vi "Trav_move_above_height.vi"(0 "Mode":T3, 1 "Extra Command String":string, 3 "Home Z":T1, 5 "New Position":sgl[](array[numeric])=[0.0, 0.0, 0.0] format="%.2f", 9 "Backlash Compensation?":bool=TRUE, 11 "Simulate/Run":T2, 12 "Row Number":i32=11, 13 "Currently on Point":i32=11, 14 "Last Part of Move?":bool=TRUE) -> (4 "Trav Position achieved":sgl[](array[numeric]) format="%.2f", 6 "Error from Traverse named":string, 15 "Error String":string)   [LabVIEW 2015]
uses:
  Trav_mode.ctl
  Controls/User_Specific_mode.ctl
  Controls/Home.ctl
  Controls/Tunnel_Coordinates.ctl
  Globals/Trav_pos_global.vi
  Globals/Extra_Commands_Global.vi
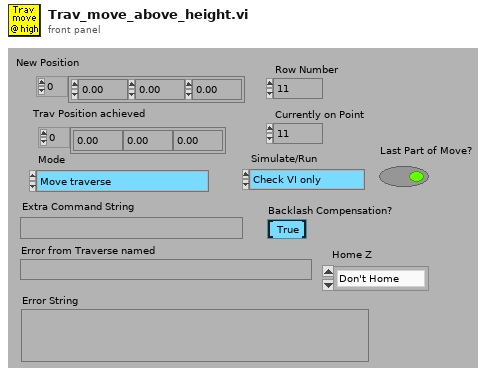
[diagram p1: front panel]
types:
  T1 = typedef "Home.ctl" = enum16{"Don't Home", "Home  +X", "Home  -X", "Home  +Y", "Home  -Y", "Home  +Z", "Home  -Z"}
  T2 = typedef "User_Specific_mode.ctl" = enum16{"Check VI only", "Run VI"}
  T3 = typedef "Trav_mode.ctl" = enum16{"Move traverse", "Read traverse position", "Teach Position"}
  T4 = typedef "Tunnel_Coordinates.ctl" = enum16{"Work in Tunnel Coordinates", "Work in Model Coordinates"}
  T5 = enum16{"To Traverse Coordinates", "To User Coordinates"}
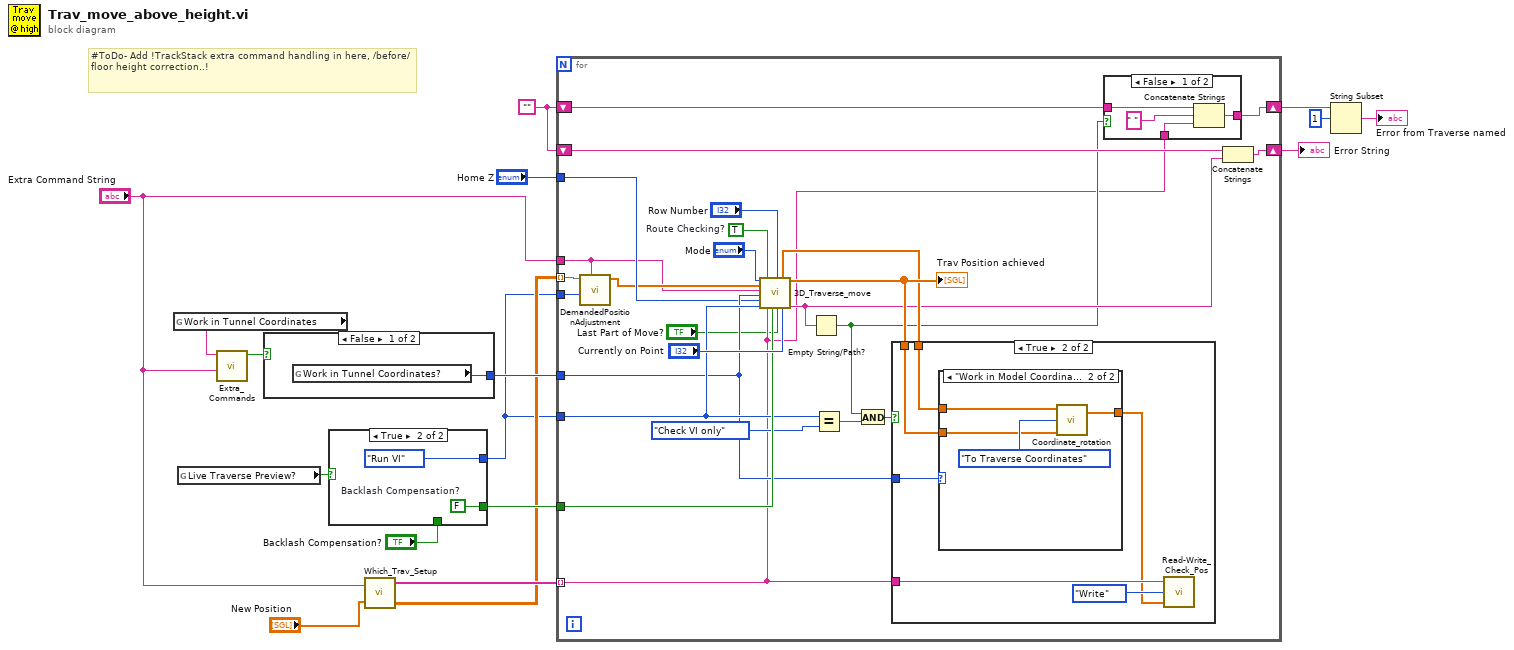
[diagram p0: block diagram]
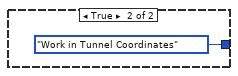
[diagram p5: hidden frame]
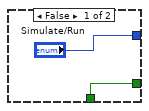
[diagram p6: hidden frame]
diagram:
  w10 = ""
  # "#ToDo- Add !TrackStack extra command handling in here, /before/ floor height correction..!"
  n1 = global read "Extra_Commands_Global.vi" "Work in Tunnel Coordinates"() -> (w14:string)
  n2 = global read "Trav_pos_global.vi" "Live Traverse Preview?"() -> (w17:bool)
  n3 = call "Extra_Commands.vi"("String to Search"="Extra Command String", "Command"=w14) -> ("Command Found"=w13:bool)  [unwired: 1 in, 4 out]
  n4 = case shown="False" w13 {
    tunnel: [w18 Tunnel_Coordinates."Work in Tunnel Coordinates" ("Work in Tunnel Coordinates?")] -> w12
    frame False {
      n5 = global read "Trav_pos_global.vi" "Work in Tunnel Coordinates?"() -> (w18:T4)
    }
    frame True {
    }
  }
  n6 = case shown="True" w17 {
    tunnel: ["Simulate/Run" User_Specific_mode."Run VI" ("Simulate/Run")] -> w1
    tunnel: [w20 w22] -> w16
    tunnel: "Backlash Compensation?" -> [w20 _]
    frame False {
    }
    frame True {
      w22 = FALSE  # Backlash Compensation?
    }
  }
  n7 = call "Which_Trav_Setup.vi"("Extra Command String"="Extra Command String", "Input Position"="New Position") -> ("Traverse Setups"=w6:string[], "Traverse Positions"=w2:sgl[][])  [unwired: 1 out]
  n8 = for {
    tunnel: w6 -> [w30] mode=indexing
    tunnel: w16 -> [w44]
    tunnel: w1 -> [w41]
    tunnel: w12 -> [w37]
    shift-right: [w34] -> w11
    shift-left: w10 -> [w35]
    shift-right: [w33] -> w9
    shift-left: w10 -> [w31]
    tunnel: "Home Z" -> [w29]
    tunnel: "Extra Command String" -> [w24]
    tunnel: w2 -> [w26] mode=indexing
    tunnel: w1 -> [w25]
    w43 = TRUE  # Route Checking?
    n9 = call "DemandedPositionAdjustment.vi"("Extra Command String"=w24, "Simulate/Run"=w25, "Demanded Position"=w26) -> ("Adjusted Position"=w27:sgl[])  [unwired: 8 in]
    n10 = call "3D_Traverse_move.vi"("Mode"="Mode", "Position"=w27, "Extra command String"=w24, "Work in Tunnel Coordinates"=w37, "Home"=w29, "Simulate/Run"=w41, "Route Checking?"=w43, "Traverse name"=w30, "Backlash Compensation?"=w44, "Row Number"="Row Number", "Last Part of Move?"="Last Part of Move?", "Currently on Point"="Currently on Point") -> ("Model:    Roll        Pitch         Yaw  (deg)"=w38:sgl[], "Trav Position achieved"=w48:sgl[], "Error String"=w36:string)  [unwired: 5 in]
    "Trav Position achieved" <- w48
    n11 = Empty String/Path?(string/path=w36) -> (empty?=w32:bool)
    n12 = Equal?(x=w41, y=User_Specific_mode."Check VI only" ("Simulate/Run")) -> (x = y?=w40:bool)
    n13 = And(x=w32, y=w40) -> (x .and. y?=w39:bool)
    n14 = case shown="True" w39 {
      tunnel: w38 -> [_ w59]
      tunnel: w48 -> [_ w58]
      tunnel: w37 -> [_ w57]
      tunnel: w30 -> [_ w55]
      frame False {
      }
      frame True {
        n15 = case shown="\"Work in Model Coordinates\"" w57 {
          tunnel: w58 -> [w60 w63]
          tunnel: [w60 w62] -> w54
          tunnel: w59 -> [_ w61]
          frame "Work in Tunnel Coordinates" {
          }
          frame "Work in Model Coordinates" {
            n16 = call "Coordinate_rotation.vi"("Roll-Pitch-Yaw"=w61, "Input Position"=w63, "Mode"=T5."To Traverse Coordinates") -> ("Output Position"=w62:sgl[])  [unwired: 2 in, 1 out]
          }
        }
        n17 = call "Read-Write_Check_Pos.vi"("Position input"=w54, "Mode"=enum16{"Read", "Write"}."Write", "Traverse Name"=w55) -> ()  [unwired: 1 out]
      }
    }
    n18 = case shown="False" w32 {
      tunnel: [w52 w53] -> w33
      tunnel: w31 -> [w51 w53]
      tunnel: w30 -> [w50 _]
      frame False {
        n19 = Concatenate Strings(w51, " " ("string"), w50) -> (w52:string)
      }
      frame True {
      }
    }
    n20 = Concatenate Strings(w35, w36) -> (w34:string)
  }
  "Error String" <- w11
  n21 = String Subset(string=w9, offset (0)=1) -> (substring=→"Error from Traverse named":string)  [unwired: 1 in]
